vi "Host-Top-Level.vi"() -> ()   [LabVIEW 2017]
uses:
  State.ctl
  <vilib>/FPGAPlugInAG/PXIe-6592R/niLvFpga_Open_PXIe-6592R.vi
  <vilib>/rvi/interface/common/dynamic/niFpgaDynamicAddResources.vi
  <vilib>/Utility/error.llb/Error Cluster From Error Code.vi
  <vilib>/rvi/errors/niLvFpgaAdjustHostInterfaceError.vi
  <vilib>/FPGAPlugInAG/Dynamic/niLvFpga_Close_Dynamic.vi
  <vilib>/rvi/interface/nirviOpenFPGA/nirviOpenFPGA.xnode
  FPGA Bitfiles/03MicroBlazeAXIS_FPGATarget_Fpga-AXI-Stream_rt9YWQdBu5Q.lvbitx
  Fpga-6592/Fpga-AXI-Stream.vi
  <vilib>/rvi/interface/nirviReadWriteControl/nirviReadWriteControl.xnode
  <vilib>/rvi/interface/nirviMethod/nirviMethod.xnode
  <vilib>/rvi/interface/nirviCloseFPGA/nirviCloseFPGA.xnode
  <vilib>/rvi/errors/niLvFpgaMergeErrorWithErrorCode.vi
  <vilib>/FPGAPlugInAG/Dynamic/niLvFpga_ReadFifo_Dynamic.vi
  <vilib>/rvi/interface/Simulation/niFpgaSimulationCallBeginRW.vi
  NiFpgaLv.dll
  <vilib>/FPGAPlugInAG/Dynamic/niLvFpga_WriteFifo_Dynamic.vi
panel:
  out "tdata_LastNonZero":u32
  out "tlast_Count":u16
  out "tvalid_Count":u16
  out "AXI_STR_RXD_tready_Count":u16
  out "tlast":bool
  out "tdata":u32
  out "tvalid":bool
  out "AXI_STR_RXD_tready":bool
  out "appended array":u32[](array[numeric])
  out "error out":errorcluster
  out "GPO 2":u32 format="%.0x"
  in  "Read all GPO":bool
  out "GPO_2":u32
  in  "GPI_1":u32
  in  "Test GPIO Write-Read":bool
  in  "Interrupt Number":fxp<+,4,4>=1.0
  out "Read Data":u32[](array[numeric]) format="%.0x"
  in  "DataToSend":u32[](array[numeric])=[240, 241, 242, 243, 244, 245]
  in  "Send":bool
  in  "Stop":bool
  in  "error in":errorcluster
  # "Send a packet of data, read the same data\necho'd back by MicroBlaze MCS"
  # "GPO 2 = GPI 1 * 2"
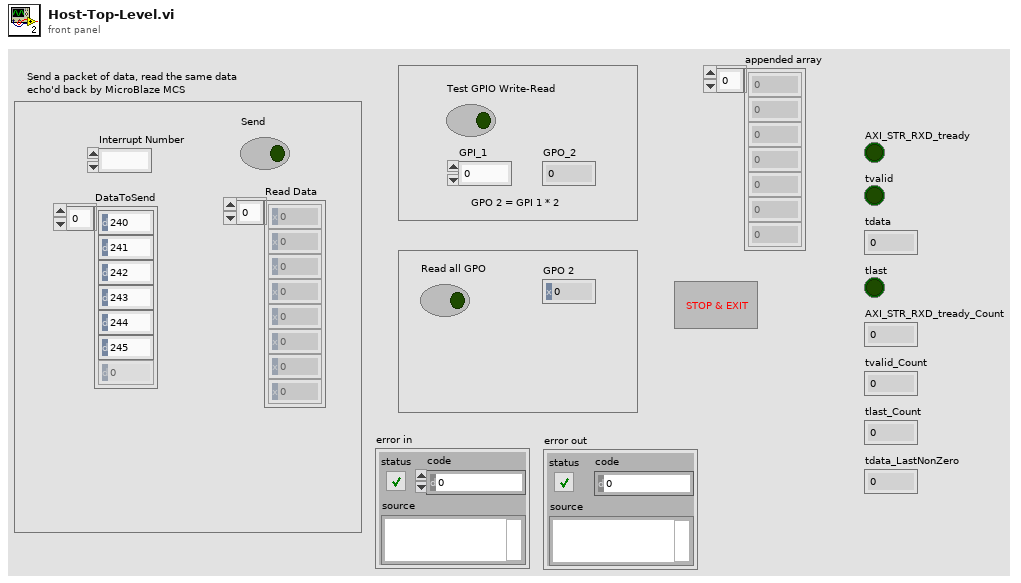
[diagram p1: front panel]
types:
  T1 = typedef "State.ctl" = enum16{"Initialize", "Idle", "Read", "Exit"}
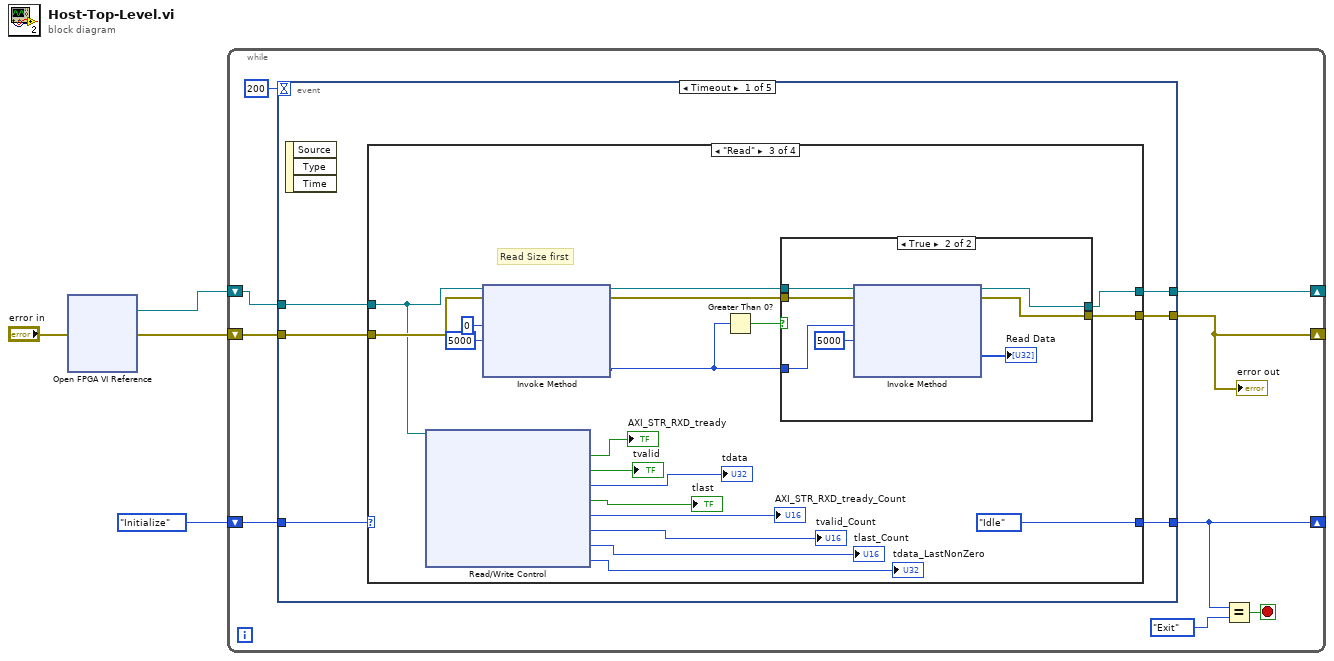
[diagram p0: block diagram]
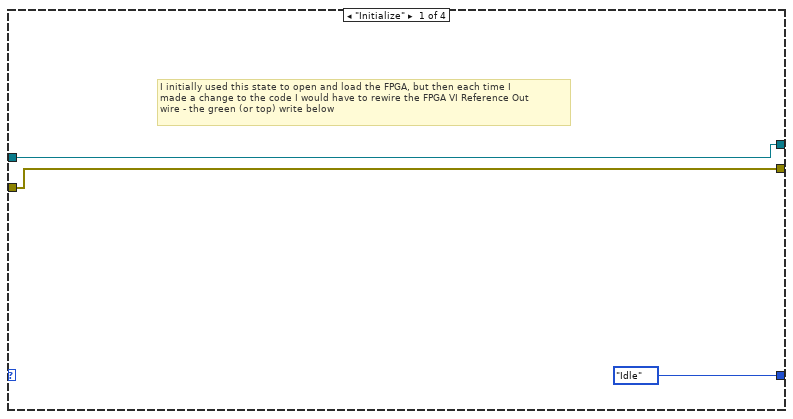
[diagram p2: hidden frame]
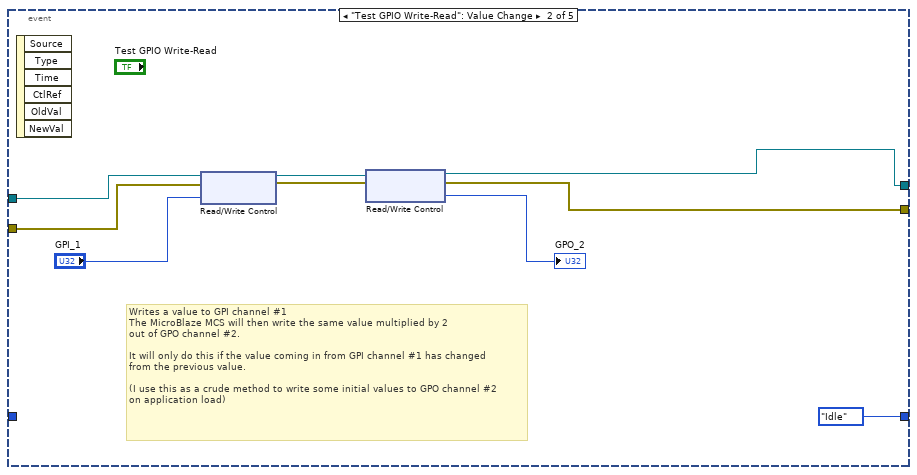
[diagram p6: hidden frame]
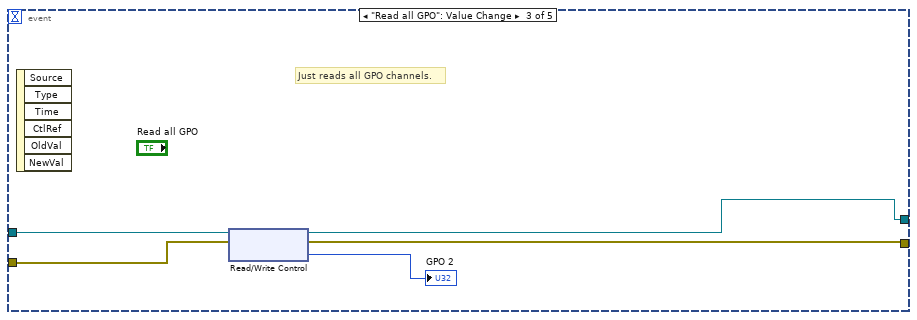
[diagram p7: hidden frame]
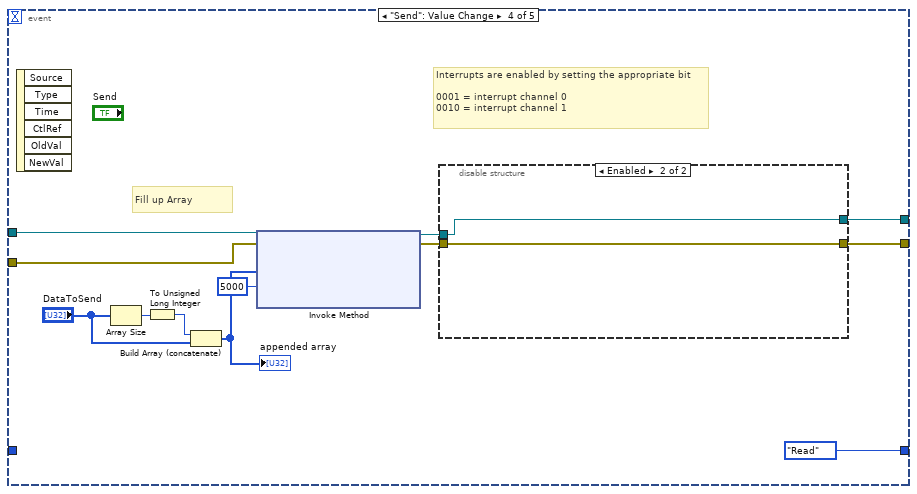
[diagram p8: hidden frame]
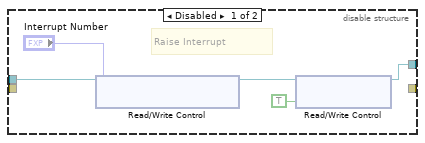
[diagram p9: hidden frame]
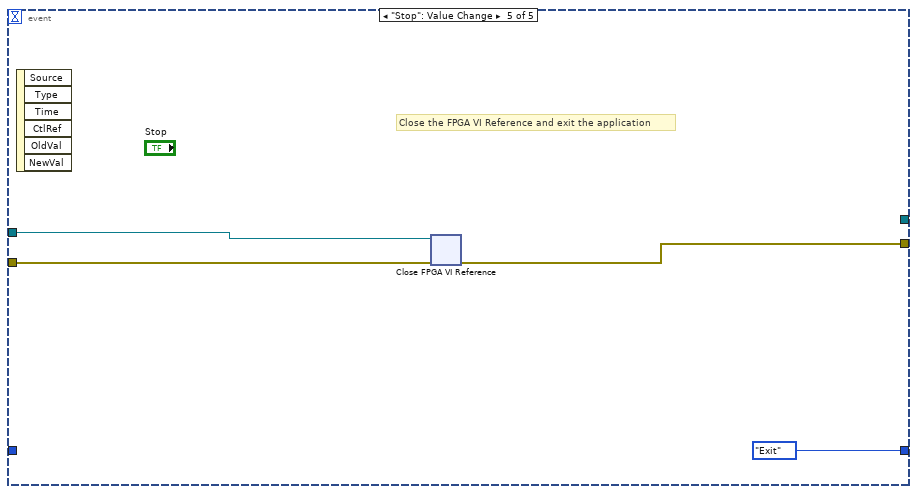
[diagram p10: hidden frame]
diagram:
  n1 = xnode "Open FPGA VI Reference"("error in"="error in") -> ("FPGA VI Reference Out"=w3:refnum<k20>, "error out"=w1:errorcluster)  [unwired: 1 in]
  n2 = while {
    shift-right: [w7] -> _
    shift-left: State."Initialize" ("Enum") -> [w13]
    shift-right: [w8] -> _
    shift-left: w1 -> [w9]
    shift-right: [w6] -> _
    shift-left: w3 -> [w5]
    stop <- w11 stop-if-true
    n3 = event shown="[0] Timeout" {
      selector: _ -> [_ _ _ _ _]
      dyn-events: _ -> [_ _ _ _ _]
      timeout: 200 -> [_ _ _ _ _]
      tunnel: [w17 State."Idle" ("Enum") _ State."Read" ("Enum") State."Exit" ("Enum")] -> w7
      tunnel: w13 -> [w16 _ _ _ _]
      tunnel: w5 -> [w15 w64 w70 w82 w93]
      tunnel: w9 -> [w19 w63 w69 w81 w92]
      tunnel: [w18 w59 w68 w72 w91] -> w8
      tunnel: [w14 w57 w66 w73 _] -> w6
      event Timeout {
        n4 = event-data() -> ()  [unwired: 1 in, 3 out]
        n5 = case shown="\"Read\"" w16 {
          selector: w16 -> [_ w24 _ w55]
          tunnel: w19 -> [w21 w25 w44 w56]
          tunnel: [w21 w25 w39 w56] -> w18
          tunnel: w15 -> [w20 w23 w35 w54]
          tunnel: [State."Idle" ("Enum") w24 State."Idle" ("Enum") w55] -> w17
          tunnel: [w20 w23 w36 w54] -> w14
          frame "Initialize" {
            # "I initially used this state to open and load the FPGA, but then each time I \nmade a change to the code I would have to rewire the FPGA VI Reference Out \nwire - the green (or top) write below"
          }
          frame "Idle", Default {
          }
          frame "Read" {
            # "Read Size first"
            n6 = xnode "Read/Write Control"("FPGA VI Reference In"=w35) -> ("AXI_STR_RXD_tready"=→"AXI_STR_RXD_tready":bool, "tvalid"=→"tvalid":bool, "tdata"=→"tdata":u32, "tlast"=→"tlast":bool, "AXI_STR_RXD_tready_Count"=→"AXI_STR_RXD_tready_Count":u16, "tvalid_Count"=→"tvalid_Count":u16, "tlast_Count"=→"tlast_Count":u16, "tdata_LastNonZero"=→"tdata_LastNonZero":u32)  [unwired: 1 in, 2 out]
            n7 = xnode "Invoke Method"("FPGA VI Reference In"=w35, "error in"=w44, "Number of Elements"=u32 0, "Timeout (ms)"=5000) -> ("FPGA VI Reference Out"=w40:refnum<k20>, "error out"=w41:errorcluster, "Elements Remaining"=w26:u32)  [unwired: 1 out]
            n8 = Greater Than 0?(x=w26) -> (x > 0?=w37:bool)
            n9 = case shown="True" w37 {
              tunnel: w41 -> [w46 w53]
              tunnel: w40 -> [w45 w52]
              tunnel: [w46 w50] -> w39
              tunnel: [w45 w49] -> w36
              tunnel: w26 -> [_ w47]
              frame False {
              }
              frame True {
                n10 = xnode "Invoke Method"("FPGA VI Reference In"=w52, "error in"=w53, "Number of Elements"=w47, "Timeout (ms)"=5000) -> ("FPGA VI Reference Out"=w49:refnum<k20>, "error out"=w50:errorcluster, "Data"=→"Read Data":u32[])  [unwired: 1 out]
              }
            }
          }
          frame "Exit" {
          }
        }
      }
      event "Test GPIO Write-Read": Value Change {
        # "Writes a value to GPI channel #1\nThe MicroBlaze MCS will then write the same value multiplied by 2\nout of GPO channel #2.\n\nIt will only do this if the value coming in from GPI channel #1 has changed\nfrom the previous value.\n\n(I use this as a crude method to write some initial values to GPO channel #2\non application load)"
        n11 = event-data() -> ()  [unwired: 1 in, 6 out]
        n12 = xnode "Read/Write Control"("FPGA VI Reference In"=w64, "error in"=w63, "GPIO1_tri_i"="GPI_1") -> ("FPGA VI Reference Out"=w58:refnum<k20>, "error out"=w61:errorcluster)
        n13 = xnode "Read/Write Control"("FPGA VI Reference In"=w58, "error in"=w61) -> ("FPGA VI Reference Out"=w57:refnum<k20>, "error out"=w59:errorcluster, "GPIO2_tri_o"=→"GPO_2":u32)
      }
      event "Read all GPO": Value Change {
        # "Just reads all GPO channels."
        n14 = event-data() -> ()  [unwired: 1 in, 6 out]
        n15 = xnode "Read/Write Control"("FPGA VI Reference In"=w70, "error in"=w69) -> ("FPGA VI Reference Out"=w66:refnum<k20>, "error out"=w68:errorcluster, "GPIO2_tri_o"=→"GPO 2":u32)
      }
      event "Send": Value Change {
        # "Interrupts are enabled by setting the appropriate bit\n\n0001 = interrupt channel 0\n0010 = interrupt channel 1"
        # "Fill up Array"
        n16 = event-data() -> ()  [unwired: 1 in, 6 out]
        n17 = Array Size(array="DataToSend") -> (size(s)=w79:i32)
        n18 = To Unsigned Long Integer(number=w79) -> (unsigned 32bit integer=w76:u32)
        n19 = Build Array (concatenate)(w76, "DataToSend") -> (w77:u32[])
        "appended array" <- w77
        n20 = xnode "Invoke Method"("FPGA VI Reference In"=w82, "error in"=w81, "Data"=w77, "Timeout (ms)"=5000) -> ("FPGA VI Reference Out"=w80:refnum<k20>, "error out"=w71:errorcluster)  [unwired: 1 out]
        n21 = disable-structure shown="Enabled" {
          disable-tunnel: w80 -> [w87 w89]
          disable-tunnel: [w83 w89] -> w73
          disable-tunnel: [_ w88] -> w72
          disable-tunnel: w71 -> [_ w88]
          frame Disabled {
            # "Raise Interrupt"
            n22 = xnode "Read/Write Control"("FPGA VI Reference In"=w87, "d_mcs_i\\INTC_Interrupt"="Interrupt Number") -> ("FPGA VI Reference Out"=w85:refnum<k20>)  [unwired: 1 in, 1 out]
            n23 = xnode "Read/Write Control"("FPGA VI Reference In"=w85, "Write Interrupt"=TRUE) -> ("FPGA VI Reference Out"=w83:refnum<k20>)  [unwired: 1 in, 1 out]
          }
          frame Enabled {
          }
        }
      }
      event "Stop": Value Change {
        # "Close the FPGA VI Reference and exit the application"
        n24 = event-data() -> ()  [unwired: 1 in, 6 out]
        n25 = xnode "Close FPGA VI Reference"("FPGA VI Reference In"=w93, "error in"=w92) -> ("error out"=w91:errorcluster)
      }
    }
    "error out" <- w8
    n26 = Equal?(x=w7, y=State."Exit") -> (x = y?=w11:bool)
  }
